vi "Dashboard Main.vi"() -> ()   [LabVIEW 2011]
uses:
  <vilib>/Rock Robotics/WPI/Camera/WPI_CameraImageSize.ctl
  <vilib>/Utility/inputDevices.llb/keyboardAcquire.vi
  Program Files (x86)/FRC Dashboard/GMXInput.dll
panel:
  in  "Tab Control":enum32{"Match Play", "Debugging"}(tab)
  out "Left":bool
  out "Elapsed Time (s)":i8
  out "Centered":bool
  out "Right":bool
  out "Camera Image":T1(plugin-control)
  in  "Mask Enable":bool=TRUE
  in  "Video Enable":bool=TRUE
  out "HIGH":bool
  out "LOW":bool
  out "Reverse-Low":bool
  out "Reverse-High":bool
  out "Right-Low":bool
  out "Right-High":bool
  out "Left-Low":bool
  out "Left-High":bool
  out "Forward-Low":bool
  out "Forward-High":bool
  out "Dashboard Datatype Warning":string="Warning: The Dashboard Datatype used by the robot project and this dashboard do not match.\nSee diagram for more details."
  out "Image Error Message":string="Timeout in Camera Communications"
  # "DRIVE"
  # "LOW"
  # "INTAKE"
  # "PNEUMATICS"
  # "SENSORS"
  # "HIGH"
  # "FORWARD"
  # "LEFT"
  # "RIGHT"
  # "REVERSE"
  # "SHOOTER"
  # "SHIFTER"
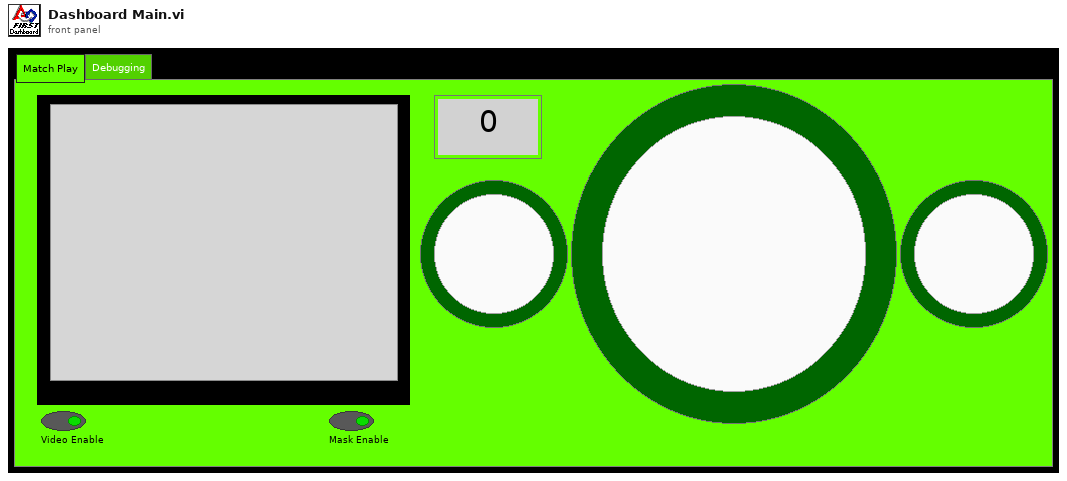
[diagram p1: front panel]
types:
  T1 = typedef "IMAQ Image.ctl" = refnum<image>
  T2 = typedef "Image Type" = u32
  T3 = typedef "WPI_CameraImageSize.ctl" = enum16{"640x480", "320x240", "160x120"}
  T4 = cluster{"fps":i32, "compression":i32, "Image Size":T3}
  T5 = enum8{"Disconnected", "E-Stop", "Disabled", "Enabled"}
  T6 = cluster{"Digital Inputs":bool[], "Digital Outputs":bool[]}
  T7 = cluster{"Competition mode":bool, "Robot Link":bool, "Autonomous":bool, "Enabled":bool, "E-Stop":bool}
  T8 = typedef "LVRectTypeDef.ctl" = cluster{"left":i16, "top":i16, "right":i16, "bottom":i16}
  T9 = enum16{"0", "1", "2", "3", "4", "5", "6", "7", "8", "9", "A", "B", "C", "D", "E", "F", "G", "H", "I", "J", "K", "L", "M", "N", "O", "P", "Q", "R", "S", "T", "U", "V", "W", "X", "Y", "Z", "F1", "F2", "F3", "F4", "F5", "F6", "F7", "F8", "F9", "F10", "F11", "F12", "F13", "F14", "F15", "ADD", "BACK", "BACKSLASH", "CAPITAL", "COMMA", "DECIMAL", "DELETE", "DIVIDE", "DOWN", "END", "EQUALS", "ESCAPE", "GRAVE (`)", "HOME", "INSERT", "LBRACKET", "LCONTROL", "LEFT", "L ALT", "LSHIFT", "LWIN", "MINUS", "MULTIPLY", "NEXT", "NUMLOCK", "NUMPAD_0", "NUMPAD_1", "NUMPAD_2", "NUMPAD_3", "NUMPAD_4", "NUMPAD_5", "NUMPAD_6", "NUMPAD_7", "NUMPAD_8", "NUMPAD_9", "PAUSE", "PERIOD", "PRIOR (PG UP)", "RBRACKET", "RCONTROL", "RETURN", "RIGHT", "R ALT", "RSHIFT", "RWIN", "SCROLL", "SEMICOLON", "SLASH", "SPACE", "SUBTRACT", "TAB", "UP", "ENTER (num pad)", "' (quote)"}
  T10 = enum16{"0", "1", "2", "3", "4", "5", "6", "7", "8", "9", "A", "B", "C", "D", "E", "F", "G", "H", "I", "J", "K", "L", "M", "N", "O", "P", "Q", "R", "S", "T", "U", "V", "W", "X", "Y", "Z", "F1", "F2", "F3", "F4", "F5", "F6", "F7", "F8", "F9", "F10", "F11", "F12", "F13", "F14", "F15", "ADD", "BACK", "BACKSLASH", "CAPITAL", "COMMA", "DECIMAL", "DELETE", "DIVIDE", "DOWN", "END", "EQUALS", "ESCAPE", "GRAVE (`)", "HOME", "INSERT", "LBRACKET", "LCONTROL", "LEFT", "L ALT", "LSHIFT", "LWIN", "MINUS", "MULTIPLY", "NEXT", "NUMLOCK", "NUMPAD_0", "NUMPAD_1", "NUMPAD_2", "NUMPAD_3", "NUMPAD_4", "NUMPAD_5", "NUMPAD_6", "NUMPAD_7", "NUMPAD_8", "NUMPAD_9", "PAUSE", "PERIOD", "PRIOR (PG UP)", "RBRACKET", "RCONTROL", "RETURN", "RIGHT", "R ALT", "RSHIFT", "RWIN", "SCROLL", "SEMICOLON", "SLASH", "SPACE", "SUBTRACT", "TAB", "UP", "ENTER (num pad)", "' (quote)"}[]
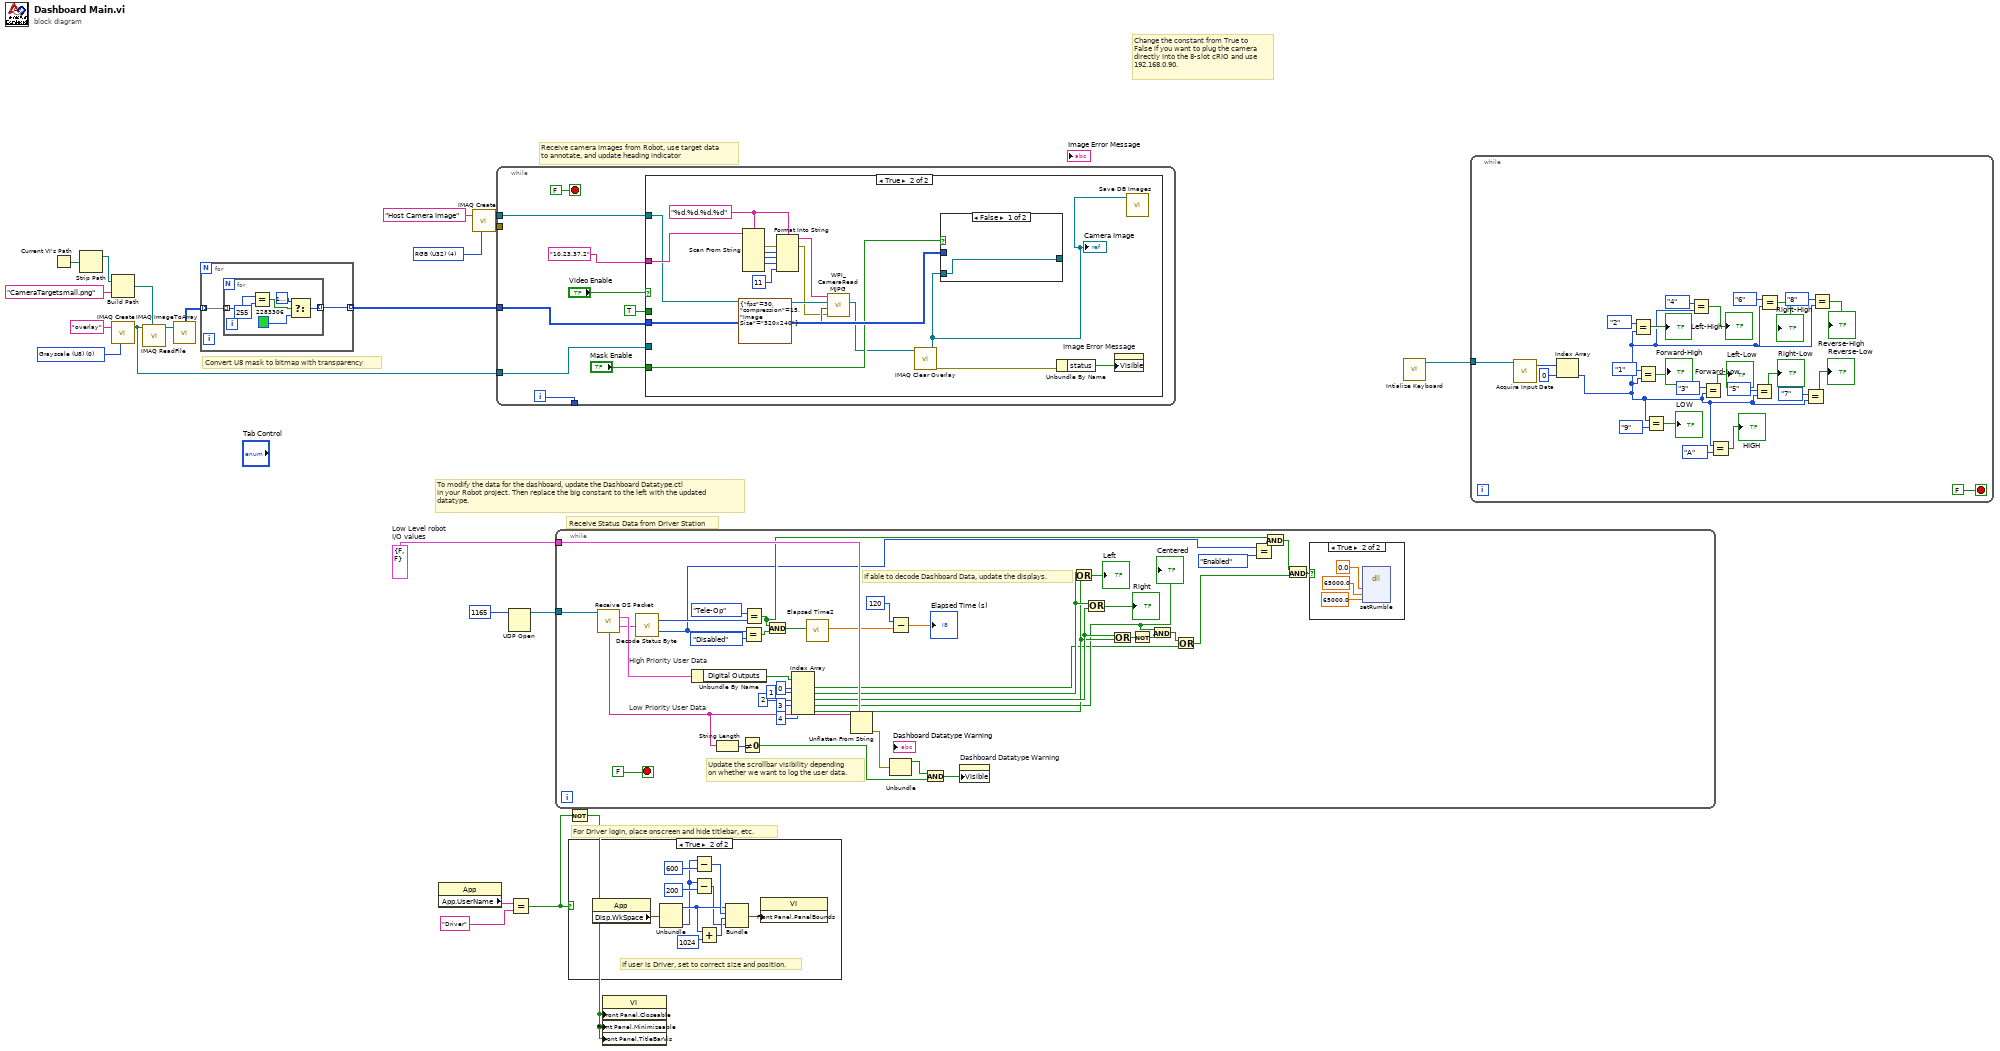
[diagram p0: block diagram]
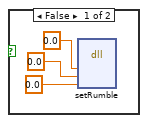
[diagram p3: hidden frame]
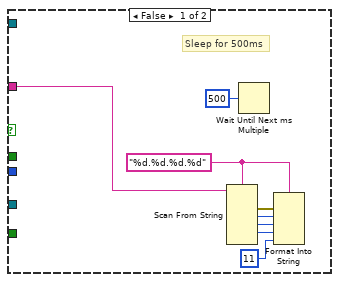
[diagram p4: hidden frame]
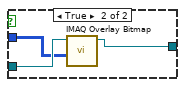
[diagram p5: hidden frame]
diagram:
  w5 = T2 0 items=["Grayscale (U8)", "Grayscale (I16)", "Grayscale (SGL)", "Complex (CSG)", "RGB (U32)", "HSL (U32)", "RGB (U64)", "Grayscale (U16)"] ("Image Type")
  w12 = cluster{bool, bool} {FALSE, FALSE}  # Low Level robot I/O values
  w20 = T2 4 items=["Grayscale (U8)", "Grayscale (I16)", "Grayscale (SGL)", "Complex (CSG)", "RGB (U32)", "HSL (U32)", "RGB (U64)"] ("Image Type")
  # "Convert U8 mask to bitmap with transparency"
  # "Change the constant from True to\nFalse if you want to plug the camera\ndirectly into the 8-slot cRIO and use\n192.168.0.90."
  # "For Driver login, place onscreen and hide titlebar, etc."
  # "To modify the data for the dashboard, update the Dashboard Datatype.ctl\nin your Robot project. Then replace the big constant to the left with the updated\ndatatype."
  # "Receive Status Data from Driver Station"
  # "Receive camera images from Robot, use target data\nto annotate, and update heading indicator"
  n1 = Current VI's Path() -> (path=w10:path)
  n2 = Strip Path(path=w10) -> (stripped path=w8:path)  [unwired: 1 out]
  n3 = Build Path(base path=w8, name or relative path="CameraTargetsmall.png") -> (appended path=w7:path)
  n4 = call "IMAQ Create"("Image Name"="overlay", "Image Type"=w5) -> ("New Image"=w2:T1)  [unwired: 3 in, 1 out]
  n5 = call "IMAQ ReadFile"("File Path"=w7, "Image"=w2) -> ("Image Out"=w3:T1)  [unwired: 5 in, 4 out]
  n6 = call "IMAQ ImageToArray"("Image"=w3) -> ("Image Pixels (U8)"=w4:u8[][])  [unwired: 3 in, 4 out]
  n7 = for {
    tunnel: w4 -> [w24] mode=indexing
    tunnel: [w23] -> w11 mode=indexing
    n8 = for {
      tunnel: w24 -> [w29] mode=indexing
      tunnel: [w30] -> w23 mode=indexing
      n9 = Equal?(x=w29, y=u8 255) -> (x = y?=w27:bool)
      n10 = Select(t=u32 16777216, s=w27, f=u32 2283306) -> (s? t:f=w30:u32)
    }
  }
  n11 = property class="App"() -> ("App.UserName"=w15:string)  [unwired: 2 in, 2 out]
  n12 = call "IMAQ Create"("Image Name"="Host Camera Image", "Image Type"=w20) -> ("New Image"=w18:T1, "error out"=w17:errorcluster)  [unwired: 2 in, 1 out]
  n13 = while {
    tunnel: w18 -> [w38]
    tunnel: w17 -> [_]
    tunnel: [w32] -> _
    tunnel: w11 -> [w34]
    tunnel: w2 -> [w33]
    i -> [w32]
    stop <- FALSE stop-if-true
    n14 = case shown="True" "Video Enable" {
      tunnel: "10.23.37.2" ("Robot IP Address") -> [w40 w56]
      tunnel: w38 -> [_ w53]
      tunnel: TRUE -> [_ _]
      tunnel: "Mask Enable" -> [_ w61]
      tunnel: w34 -> [_ w62]
      tunnel: w33 -> [_ _]
      frame False {
        w41 = "%d.%d.%d.%d" ("format string")
        # "Sleep for 500ms"
        n15 = Scan From String(format string=w41, input string=w40) -> (error out=w43:errorcluster, output 1=w44:i32, output 2=w45:i32, output 3=w46:i32)  [unwired: 2 in, 7 out]
        n16 = Wait Until Next ms Multiple(millisecond multiple=u32 500) -> ()  [unwired: 1 out]
        n17 = Format Into String(format string=w41, error in=w43, w44, w45, w46, 11 ("IP Suffix:")) -> ()  [unwired: 1 in, 2 out]
      }
      frame True {
        w54 = "%d.%d.%d.%d" ("format string")
        n18 = Scan From String(format string=w54, input string=w56) -> (error out=w57:errorcluster, output 1=w58:i32, output 2=w59:i32, output 3=w60:i32)  [unwired: 2 in, 7 out]
        n19 = Format Into String(format string=w54, error in=w57, w58, w59, w60, 11 ("IP Suffix:")) -> (resulting string=w49:string, error out=w50:errorcluster)  [unwired: 1 in]
        n20 = call <vilib>:"WPI_CameraRead MJPG.vi"("error in"=w50, "Camera Settings"=T4 {"fps"=30, "compression"=15, "Image Size"=enum."320x240"}, "Image"=w53, "address"=w49) -> ("Image Out"=w51:T1)  [unwired: 6 in, 1 out]
        n21 = call "IMAQ Clear Overlay"("Image"=w51) -> ("error out"=w63:errorcluster, "Image Out"=w48:T1)  [unwired: 2 in, 7 out]
        "Camera Image" <- w48
        n22 = case shown="False" w61 {
          tunnel: w62 -> [_ w66]
          tunnel: w48 -> [w65 w67]
          tunnel: [w65 w68] -> _
          frame False {
          }
          frame True {
            n23 = call "IMAQ Overlay Bitmap"("Bitmap"=w66, "Image"=w67) -> ("Image Out"=w68:T1)  [unwired: 8 in, 1 out]
          }
        }
        n24 = Unbundle By Name(w63) -> ("status"=w64:bool)
        n25 = property on="Image Error Message" class="Str"("Visible"=w64) -> ()  [unwired: 2 in, 2 out]
        n26 = call "Save DB Images.vi"("Image"=w48) -> ()  [unwired: 2 in, 1 out]
      }
    }
  }
  n27 = UDP Open(11:u16 1165 ("port")) -> (port=w21:refnum<k16>)  [unwired: 2 in, 4 out]
  n28 = Equal?(x=w15, y="Driver") -> (x = y?=w14:bool)
  n29 = while {
    tunnel: w21 -> [w109]
    tunnel: w12 -> [w108]
    stop <- FALSE stop-if-true
    # "High Priority User Data"
    # "Low Priority User Data"
    # "Update the scrollbar visibility depending\non whether we want to log the user data."
    # "If able to decode Dashboard Data, update the displays."
    n30 = call "Receive DS Packet.vi"("Recv Socket"=w109) -> ("Driver Station"=w102:T6, "Status"=w86:T7, "Low Priority User Data"=w98:string)  [unwired: 1 in, 11 out]
    n31 = call "Decode Status Byte.vi"("Status Byte"=w86) -> ("Mode"=w84:enum8{"Tele-Op", "Auto", ""}, "Status"=w75:T5)
    n32 = Unbundle By Name(w102) -> ("Digital Outputs"=w101:bool[])
    n33 = String Length(string=w98) -> (length=w103:i32)
    n34 = Not Equal To 0?(x=w103) -> (x != 0?=w105:bool)
    n35 = Equal?(x=w75, y=T5."Disabled" ("Status")) -> (x = y?=w82:bool)
    n36 = Equal?(x=enum8{"Tele-Op", "Auto", ""}."Tele-Op" ("Mode"), y=w84) -> (x = y?=w77:bool)
    n37 = And(x=w77, y=w82) -> (x .and. y?=w81:bool)
    n38 = Index Array(array=w101, index #1=0 ("index"), index #2=1 ("index"), index #3=2 ("index"), index #4=3 ("index"), index #5=4 ("index")) -> (element #1=w69:bool, element #2=w94:bool, element #3=w91:bool, element #4=w87:bool, element #5=w90:bool)
    "Centered" <- w87
    n39 = call "Elapsed Time2"("Reset"=w81) -> ("Elapsed Time (s)"=w80:dbl)  [unwired: 11 in, 7 out]
    n40 = Unflatten From String(type=w108, binary string=w98) -> (error out=w107:errorcluster)  [unwired: 1 in, 4 out]
    n41 = Subtract(x=120, y=w80) -> (x-y=→"Elapsed Time (s)":dbl)
    n42 = Unbundle(w107) -> ("status"=w104:bool)  [unwired: 2 out]
    n43 = And(x=w104, y=w105) -> (x .and. y?=w106:bool)
    n44 = property on="Dashboard Datatype Warning" class="Str"("Visible"=w106) -> ()  [unwired: 2 in, 2 out]
    n45 = Or(x=w94, y=w90) -> (x .or. y?=→"Left":bool)
    n46 = Or(x=w94, y=w91) -> (x .or. y?=→"Right":bool)
    n47 = Or(x=w91, y=w90) -> (x .or. y?=w89:bool)
    n48 = Not(x=w89) -> (.not. x?=w88:bool)
    n49 = And(x=w87, y=w88) -> (x .and. y?=w70:bool)
    n50 = Or(x=w70, y=w69) -> (x .or. y?=w73:bool)
    n51 = Equal?(x=w75, y=T5."Enabled" ("Status")) -> (x = y?=w74:bool)
    n52 = And(x=w77, y=w74) -> (x .and. y?=w71:bool)
    n53 = And(x=w71, y=w73) -> (x .and. y?=w72:bool)
    n54 = case shown="True" w72 {
      frame False {
        n55 = dll-call lib="C:/Program Files (x86)/FRC Dashboard/GMXInput.dll" fn="setRumble"("Index"=0.0, "leftMotorSpeed"=0.0 ("Index"), "rightMotorSpeed"=0.0 ("Index")) -> ()  [unwired: 7 in, 2 out]
      }
      frame True {
        n56 = dll-call lib="C:/Program Files (x86)/FRC Dashboard/GMXInput.dll" fn="setRumble"("Index"=0.0, "leftMotorSpeed"=65000.0 ("Index"), "rightMotorSpeed"=65000.0 ("Index")) -> ()  [unwired: 7 in, 2 out]
      }
    }
  }
  n57 = Not(x=w14) -> (.not. x?=w13:bool)
  n58 = case shown="True" w14 {
    frame False {
    }
    frame True {
      # "If user is Driver, set to correct size and position."
      n59 = property class="App"() -> ("Disp.WkSpace"=w126:T8)  [unwired: 2 in, 2 out]
      n60 = Unbundle(w126) -> ("left"=w121:i16, "bottom"=w117:i16)  [unwired: 2 out]
      n61 = Subtract(x=w117, y=600) -> (x-y=w123:i32)
      n62 = Subtract(x=w117, y=200) -> (x-y=w118:i32)
      n63 = Add(x=w121, y=1024) -> (x+y=w122:i32)
      n64 = Bundle("left"=w121, w123, w122, w118) -> (w125:cluster{"left":i16, i32, i32, i32})  [unwired: 1 out]
      n65 = property class="VI"("Front Panel.PanelBounds"=w125) -> ()  [unwired: 2 in, 2 out]
    }
  }
  n66 = property class="VI"("Front Panel.Closeable"=w13, "Front Panel.Minimizeable"=w13, "Front Panel.TitleBarVis"=w13) -> ()  [unwired: 2 in, 2 out]
  n67 = call <vilib>:"Intialize Keyboard.vi"() -> ("device ID"=w1:refnum<k1>)  [unwired: 10 in, 1 out]
  n68 = while {
    tunnel: w1 -> [w130]
    stop <- FALSE stop-if-true
    n69 = call-poly <vilib>:"Acquire Input Data.vi"("device ID"=w130) -> ("keys pressed"=w131:T10)  [unwired: 16 in, 2 out]
    n70 = Index Array(array=w131, index=0) -> (element=w129:T9)
    n71 = Equal?(x=T9."2" ("element"), y=w129) -> (x = y?=→"Forward-High":bool)
    n72 = Equal?(x=T9."1" ("element"), y=w129) -> (x = y?=→"Forward-Low":bool)
    n73 = Equal?(x=w129, y=T9."9" ("element")) -> (x = y?=→"LOW":bool)
    n74 = Equal?(x=T9."4" ("element"), y=w129) -> (x = y?=→"Left-High":bool)
    n75 = Equal?(x=T9."3" ("element"), y=w129) -> (x = y?=→"Left-Low":bool)
    n76 = Equal?(x=w129, y=T9."A" ("element")) -> (x = y?=→"HIGH":bool)
    n77 = Equal?(x=T9."5" ("element"), y=w129) -> (x = y?=→"Right-Low":bool)
    n78 = Equal?(x=T9."6" ("element"), y=w129) -> (x = y?=→"Right-High":bool)
    n79 = Equal?(x=T9."7" ("element"), y=w129) -> (x = y?=→"Reverse-Low":bool)
    n80 = Equal?(x=T9."8" ("element"), y=w129) -> (x = y?=→"Reverse-High":bool)
  }
